vi "SendResults.vi"(8 "error in (no error)":errorcluster, 10 "Result Json":string, 11 "Inference in":refnum<class "Inference.lvclass">) -> (0 "error out":errorcluster, 3 "Inference out":refnum<class "Inference.lvclass">)   [LabVIEW 2019, in "Inference.lvlib" / "Inference.lvclass"]
uses:
  Inference.lvclass
  C:/Program Files/National Instruments/LabVIEW 2019/vi.lib/ActorFramework/Actor/Actor.lvclass
  <vilib>/ActorFramework/Actor/Actor.lvclass/Actor.ctl
  Inference.lvclass/Inference.ctl
  Inference Messages/Result Msg/Result Msg.lvclass/Result Msg.ctl
  <vilib>/ActorFramework/Message Enqueuer/Message Enqueuer.lvclass/Message Enqueuer.ctl
  <vilib>/ActorFramework/Message Enqueuer/Enqueue.vi
  Inference Messages/Result Msg/Result Msg.lvclass
  C:/Program Files/National Instruments/LabVIEW 2019/vi.lib/ActorFramework/Message/Message.lvclass
  <vilib>/ActorFramework/Message Priority Queue/Priority Enqueue.vi
  <vilib>/ActorFramework/Message Enqueuer/Message Enqueuer.lvclass
  <vilib>/ActorFramework/Actor/Actor.lvclass
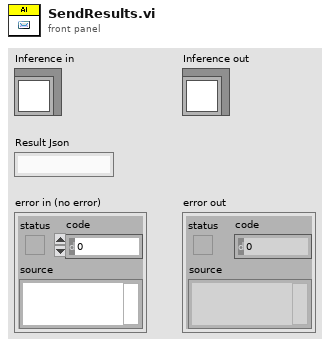
[diagram p1: front panel]
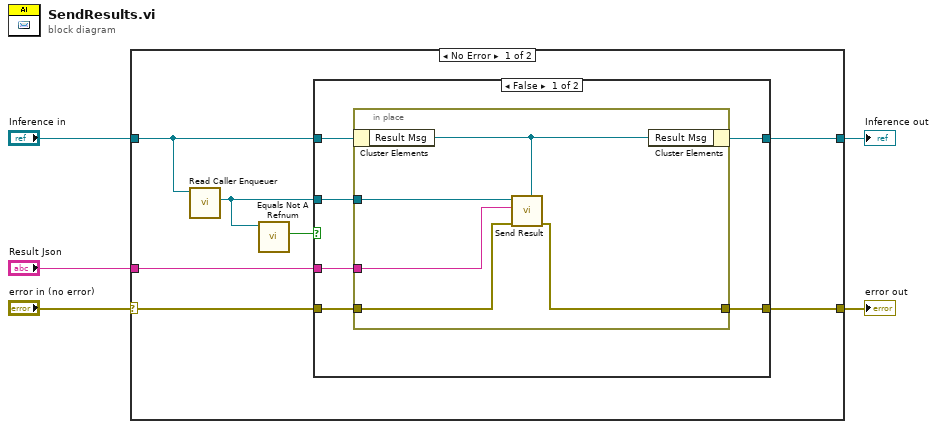
[diagram p0: block diagram]
diagram:
  n1 = case shown="No Error" "error in (no error)" {
    selector: "error in (no error)" -> [w8 w27]
    tunnel: [w7 w27] -> w4
    tunnel: [w6 w26] -> w2
    tunnel: "Inference in" -> [w10 w26]
    tunnel: "Result Json" -> [w11 _]
    frame No Error {
      n2 = call <vilib>:"Read Caller Enqueuer.vi"("Actor"=w10) -> ("Caller Enqueuer"=w9:refnum<class "Message Enqueuer.lvclass">)  [unwired: 10 in]
      n3 = call <vilib>:"Equals Not A Refnum.vi"("Message Enqueuer"=w9) -> ("Not a refnum?"=w12:bool)  [unwired: 10 in]
      n4 = case shown="False" w12 {
        tunnel: w11 -> [w16 _]
        tunnel: w10 -> [w18 w25]
        tunnel: w9 -> [w17 _]
        tunnel: w8 -> [w15 w24]
        tunnel: [w14 w24] -> w7
        tunnel: [w13 w25] -> w6
        frame False {
          n5 = in-place {
            in-place-border: w17 -> [w23]
            in-place-border: w16 -> [w22]
            in-place-border: w15 -> [w21]
            in-place-border: [w20] -> w14
            n6 = in-place-cluster #1(w18) -> ("Result Msg"=w19:refnum<class "Result Msg.lvclass">)
            n7 = call "Send Result.vi"("Message Type"=w19, "error in (no error)"=w21, "Json Result"=w22, "Message Enqueuer"=w23) -> ("error out"=w20:errorcluster)  [unwired: 6 in, 1 out]
            n8 = in-place-cluster #1("Result Msg"=w19) -> (w13:refnum<class "Inference.lvclass">)
          }
        }
        frame True {
        }
      }
    }
    frame Error {
    }
  }
  "error out" <- w4
  "Inference out" <- w2
